vi "MinDistanceToSegmentwAng.vi"(9 "Segment Point 2":T1 {"North" format="%#_10f"; "East" format="%#_8f"}, 10 "Segment Point 1":T1 {"North" format="%#_10f"; "East" format="%#_8f"}, 11 "Boat Point":T1 {"North" format="%#_10f"; "East" format="%#_8f"}) -> (0 "Closest point to boat":T1 {"North" format="%#_10f"; "East" format="%#_8f"}, 1 "Angle to Obstacle, Trig Abs (deg)":dbl, 2 "Angle to Obstacle, Trig Abs (rad)":dbl(knob), 3 "Distance between boat and segment":dbl)   [LabVIEW 2013, in "Obstacle.lvclass"]
doc: "Takes in a segment, and a boat point, and returns both the minimal distance between the segment and the boat and the angle to the segment or the nearest point.\n\nEric Schneider, August 2014"
uses:
  Obstacle.lvclass
  Data/TypeDefs/UTM Location.ctl
  <vilib>/Analysis/baseanly.llb/Real Dot Product.vi
  Utilities/Math/Angles/Angle/Angle.lvclass
  <vilib>/Analysis/NI_AALBase.lvlib
panel:
  out "t":dbl
  out "Closest point on line":T2
  out "l2":dbl format="%.2f"
  # "INPUT"
  # "CALCULATION"
  # "OUTPUT"
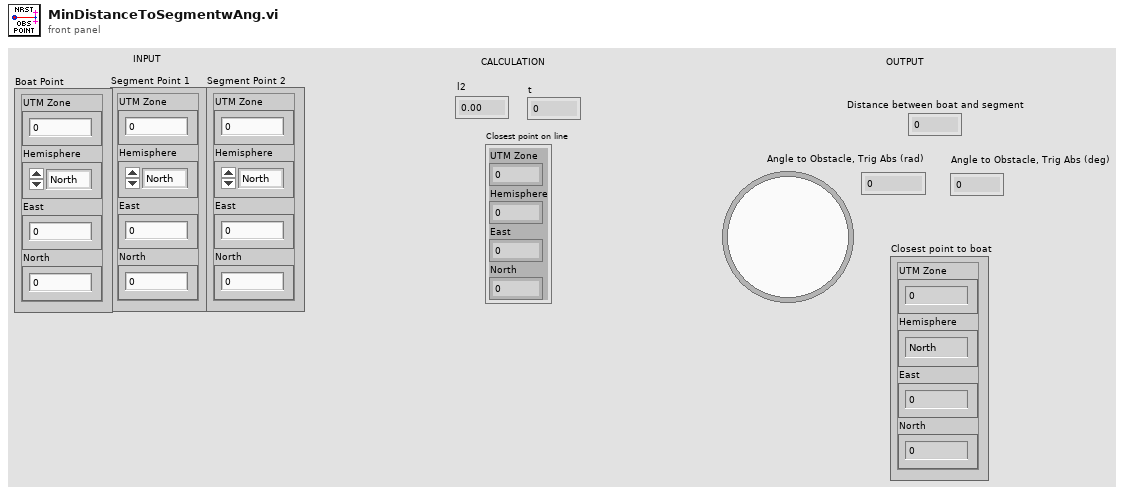
[diagram p1: front panel]
types:
  T1 = typedef "UTM Location.ctl" = cluster{"UTM Zone":dbl, "Hemisphere":enum16{"North", "South"}, "East":dbl, "North":dbl}
  T2 = cluster{"UTM Zone":dbl, "Hemisphere":dbl, "East":dbl, "North":dbl}
  T3 = cluster{"UTM Zone":dbl, "Hemisphere":u16, "East":dbl, "North":dbl}
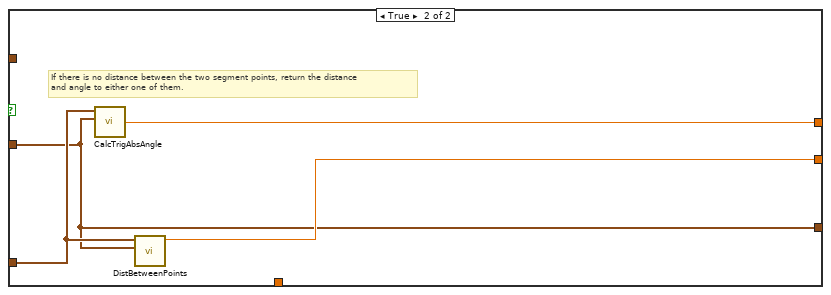
[diagram p4: hidden frame]
diagram:
  # "The math here is a little complicated. Go to http://stackoverflow.com/questions/849211/shortest-distance-between-a-point-and-a-line-segment for the explanation"
  # "Law of cosines would have been better to use in retrospect"
  # "There may be a failure case where the subtraction of absolute angles fails when done across zero, haven't been able to find it"
  # "Why the distance works, acute case:\nthe difference of the abs angles is the the angle from the segment to the boat from point 2\nthe hyp of that interior triangle is the distance between them\nsin(x) times that hyp is the opp length from the boat to the segment\nObtuse case: gets distance to obtuse angle vertex\n\nWhy the angle works for the acute case:\nCalcs the line perpendicular to the segment line, adds or subtracts pi/2 based on the relative\nabs angles of the segment and the boat.\n\nAngle for obtuse case: abs angle from obtuse angle vertex \n\nNote: Obtuse triangle only relevant when a segment point is an obtuse vertex."
  n1 = call "Initialize.vi"() -> ()  [unwired: 10 in, 2 out]
  n2 = call "DistBetweenPoints.vi"("UTM Location 2"="Segment Point 2", "UTM Location 1"="Segment Point 1") -> ("Distance from 1 to 2"=w15:dbl)  [unwired: 9 in]
  n3 = Square(x=w15) -> (x^2=w8:dbl)
  "l2" <- w8
  n4 = Equal To 0?(x=w8) -> (x = 0?=w14:bool)
  n5 = case shown="False" w14 {
    tunnel: "Boat Point" -> [w20 w52]
    tunnel: "Segment Point 2" -> [w19 w51]
    tunnel: [w17 w54] -> w13
    tunnel: [w18 w53] -> w11
    tunnel: "Segment Point 1" -> [w27 _]
    tunnel: w8 -> [w30 _]
    tunnel: [w16 w51] -> w7
    frame False {
      n6 = Subtract(x=w20, y=w27) -> (x-y=w38:T3)
      n7 = Subtract(x=w19, y=w27) -> (x-y=w28:T3)
      n8 = Unbundle By Name(w38) -> ("East"=w36:dbl, "North"=w37:dbl)
      n9 = Unbundle By Name(w28) -> ("East"=w34:dbl, "North"=w35:dbl)
      n10 = Build Array(w36, w37) -> (w33:dbl[])
      n11 = Build Array(w34, w35) -> (w32:dbl[])
      n12 = call-poly <vilib>:"Dot Product.vi"("Y Vector"=w32, "X Vector"=w33) -> ("X * Y"=w31:dbl)  [unwired: 1 out]
      n13 = Divide(x=w31, y=w30) -> (x/y=w26:dbl)
      "t" <- w26
      n14 = Less Than 0?(x=w26) -> (x < 0?=w29:bool)
      n15 = Greater?(x=w26, y=1.0) -> (0:w25:bool)
      n16 = case shown="False" w29 {
        tunnel: w28 -> [w47 _]
        tunnel: w26 -> [w46 _]
        tunnel: w27 -> [w45 w49]
        tunnel: w20 -> [w44 w50]
        tunnel: [w44 w50] -> w23
        tunnel: [w43 w49] -> w21
        frame False {
          n17 = Multiply(x=w46, y=w47) -> (x*y=w48:T2)
          n18 = Add(x=w45, y=w48) -> (x+y=w43:T2)
          "Closest point on line" <- w43
        }
        frame True {
          # "If t<0, go straight from the boat to segment point 1"
        }
      }
      n19 = case shown="True" w25 {
        tunnel: [w40 w42] -> w22
        tunnel: w23 -> [w40 _]
        tunnel: w21 -> [w39 _]
        tunnel: [w39 w41] -> w16
        tunnel: w20 -> [_ w42]
        tunnel: w19 -> [_ w41]
        frame False {
        }
        frame True {
          # "If t>1, go straight from the boat to segment point 2"
        }
      }
      n20 = call "DistBetweenPoints.vi"("UTM Location 2"=w16, "UTM Location 1"=w22) -> ("Distance from 1 to 2"=w17:dbl)  [unwired: 9 in]
      n21 = call "CalcTrigAbsAngle.vi"("Point 2"=w16, "Point 1"=w22) -> ("Angle between points (rad)"=w18:dbl)  [unwired: 8 in, 1 out]
    }
    frame True {
      # "If there is no distance between the two segment points, return the distance\nand angle to either one of them."
      n22 = call "CalcTrigAbsAngle.vi"("Point 2"=w51, "Point 1"=w52) -> ("Angle between points (rad)"=w53:dbl)  [unwired: 8 in, 1 out]
      n23 = call "DistBetweenPoints.vi"("UTM Location 2"=w51, "UTM Location 1"=w52) -> ("Distance from 1 to 2"=w54:dbl)  [unwired: 9 in]
    }
  }
  "Distance between boat and segment" <- w13
  "Angle to Obstacle, Trig Abs (rad)" <- w11
  n24 = Unbundle By Name(w7) -> ("UTM Zone"=w5:dbl, "Hemisphere"=w4:dbl, "East"=w3:dbl, "North"=w2:dbl)
  n25 = expression code="(x/pi)*180.0" "radians to degrees"(w11) -> (→"Angle to Obstacle, Trig Abs (deg)":dbl)
  n26 = Bundle By Name(cluster="Boat Point", "UTM Zone"=w5, "Hemisphere"=w4, "East"=w3, "North"=w2) -> (→"Closest point to boat":T1)
